vi "test for loop autoindexing.vi"() -> ()   [LabVIEW 2010]
panel:
  out "output2":u16[][](array[numeric])
  out "output 1":u16[][](array[numeric])
  out "loop array":u16[][](array[numeric])
  in  "2D array 2":u16[][](array[numeric])=[[3, 4], [5, 6]]
  in  "2D array 1":u16[][](array[numeric])=[[0, 1], [2, 3]]
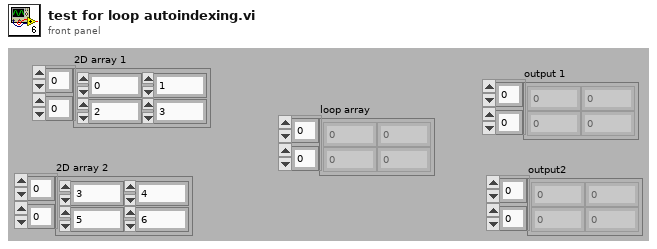
[diagram p1: front panel]
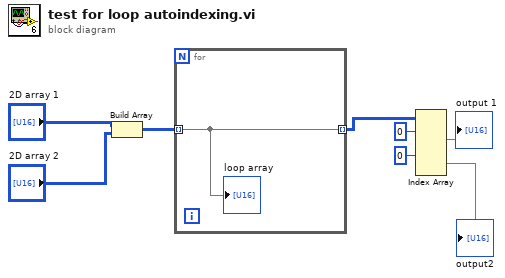
[diagram p0: block diagram]
diagram:
  n1 = Build Array("2D array 1", "2D array 2") -> (w6:u16[][][])
  n2 = for {
    tunnel: w6 -> [w9] mode=indexing
    tunnel: [w9] -> w5 mode=indexing
    "loop array" <- w9
  }
  n3 = Index Array(array=w5, index (dim 0) #1=0 ("index (page)"), index (dim 0) #2=0 ("index (page)")) -> (element #1=→"output 1":u16[][], element #2=→"output2":u16[][])  [unwired: 4 in]
